vi "Clear Report.vi"(0 "report in":refnum<class "ooWriter.lvclass">, 11 "error in (no error)":errorcluster) -> (4 "report out":refnum<class "ooWriter.lvclass">, 15 "error out":errorcluster)   [LabVIEW 2009, in "ooWriter.lvclass"]
doc: "Clears all text, headers, footers, and formatting information from the report."
uses:
  ooWriter.lvclass
  C:/Projets/LAVAG/OpenOfficeRGT/AODL/DLLs/AODL.dll
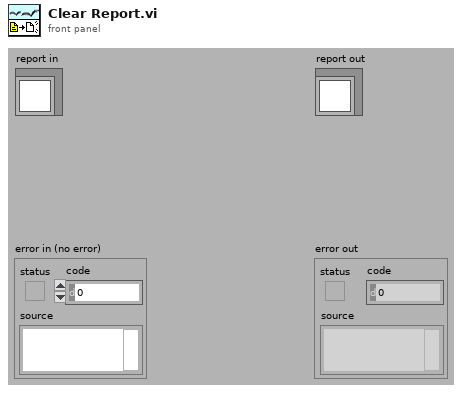
[diagram p1: front panel]
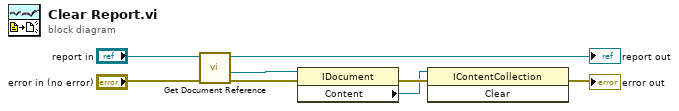
[diagram p0: block diagram]
diagram:
  n1 = call-dynamic "Get Document Reference.vi"("error in (no error)"="error in (no error)", "ooDocument in"="report in") -> ("error out"=w1:errorcluster, "Document"=w5:refnum<k24>, "ooDocument out"=→"report out":refnum<class "ooWriter.lvclass">)  [unwired: 7 in]
  n2 = property class="IDocument"(reference=w5, error in=w1) -> (error out=w7:errorcluster, "Content"=w6:refnum<k24>)  [unwired: 1 out]
  n3 = invoke class="IContentCollection" method="Clear"(reference=w6, error in=w7) -> (error out=→"error out":errorcluster)  [unwired: 1 in, 2 out]
